vi "MH_RateDatAvg.vi"(0 "Rate Data":i32[][](array[numeric]), 1 "ClearRef":refnum<vi>, 3 "Avg ref":refnum<vi>, 5 "Count Rates":i32[](array[numeric]), 9 "RateAvg Data":i32[][](array[numeric]), 11 "error in (no error)":errorcluster caption="entrée d'erreur (pas d'erreur)", 12 "Avg Val":i32) -> (4 "Rate Data Out":i32[][](array[numeric]), 6 "Data":cluster{dbl, dbl, dbl, dbl}[](array[cluster]), 10 "RateAvg Data Out":i32[][](array[numeric]) format="%.2f", 13 "ValAvg":i32[](array[numeric]), 14 "Avg Val Out":i32, 15 "error out":errorcluster caption="sortie d'erreur")   [LabVIEW 2019]
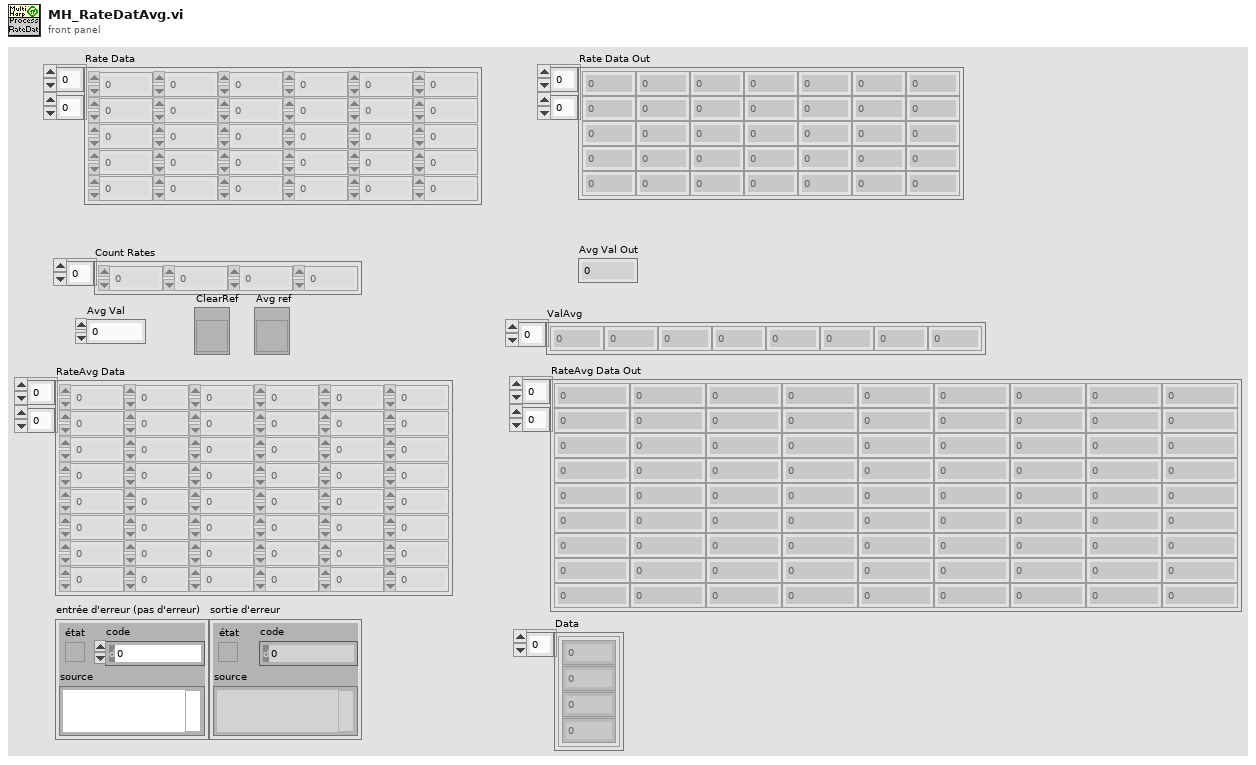
[diagram p1: front panel]
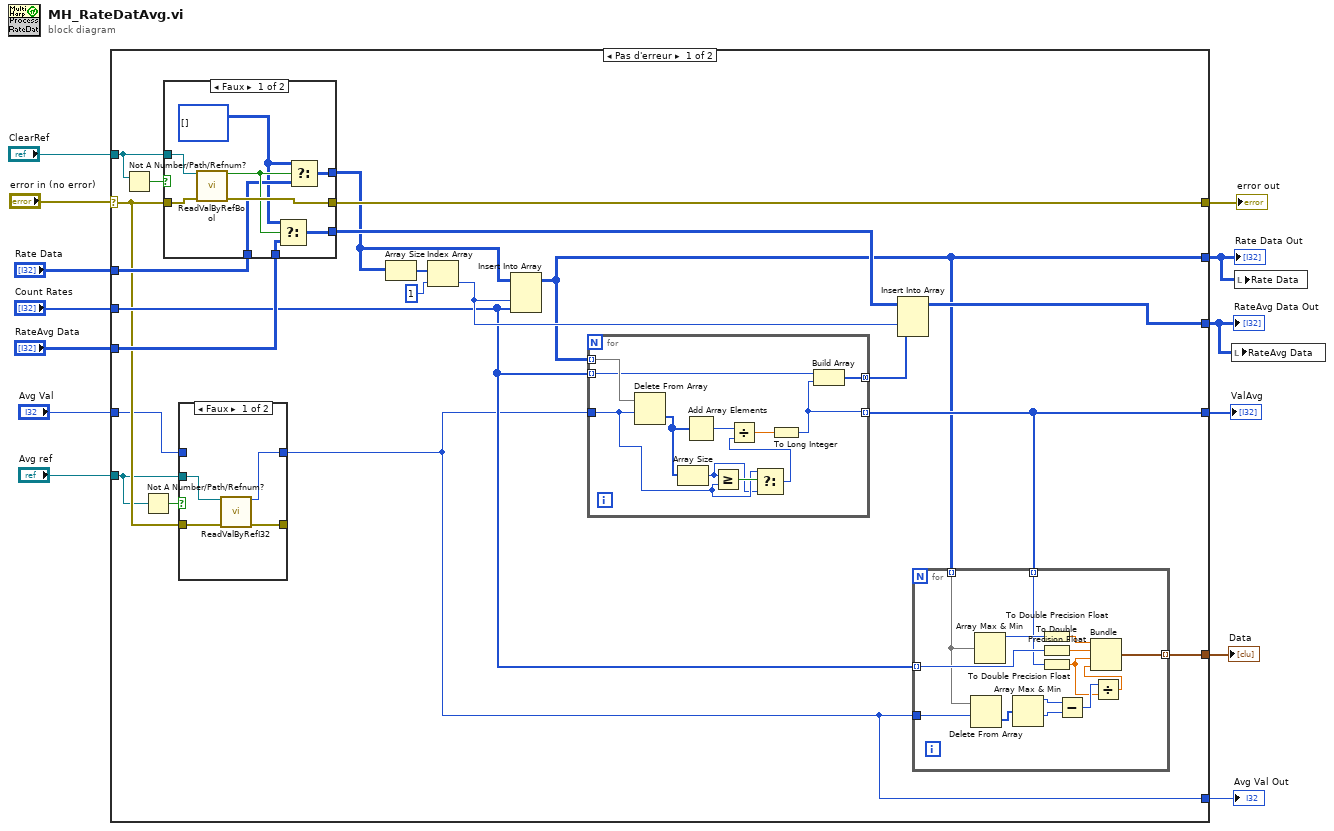
[diagram p0: block diagram]
diagram:
  n1 = case shown="Pas d'erreur" "error in (no error)" {
    selector: "error in (no error)" -> [w21 w80]
    tunnel: "Avg Val" -> [w18 _]
    tunnel: [w16 w79] -> w2
    tunnel: "Rate Data" -> [w26 w79]
    tunnel: "Count Rates" -> [w23 _]
    tunnel: "RateAvg Data" -> [w27 w78]
    tunnel: [w22 w78] -> w1
    tunnel: [w17 _] -> w9
    tunnel: [w30 w80] -> w7
    tunnel: "ClearRef" -> [w28 _]
    tunnel: "Avg ref" -> [w20 _]
    tunnel: [w15 _] -> w4
    tunnel: [w14 _] -> w3
    frame No Error {
      n2 = Not A Number/Path/Refnum?(number/path/refnum=w28) -> (NaN/Path/Refnum?=w29:bool)
      n3 = Not A Number/Path/Refnum?(number/path/refnum=w20) -> (NaN/Path/Refnum?=w19:bool)
      n4 = case shown="Faux" w29 {
        tunnel: w21 -> [w63 w66]
        tunnel: [w62 w66] -> w30
        tunnel: w28 -> [w61 _]
        tunnel: w27 -> [w58 w65]
        tunnel: w26 -> [w59 w64]
        tunnel: [w57 w65] -> w25
        tunnel: [w56 w64] -> w24
        frame False {
          w55 = i32[][] [] ("cas vrai")
          n5 = call <userlib>:"ReadValByRefBool.vi"("Control Ref"=w61, "error in"=w63) -> ("Valeur"=w60:bool, "error out"=w62:errorcluster)  [unwired: 12 in]
          n6 = Select(t=w55, s=w60, f=w58) -> (s? t:f=w57:i32[][])
          n7 = Select(t=w55, s=w60, f=w59) -> (s? t:f=w56:i32[][])
        }
        frame True {
        }
      }
      n8 = case shown="Faux" w19 {
        tunnel: w21 -> [w38 w40]
        tunnel: [w36 w40] -> _
        tunnel: w20 -> [w37 _]
        tunnel: w18 -> [_ w39]
        tunnel: [w35 w39] -> w14
        frame False {
          n9 = call <userlib>:"ReadValByRefI32.vi"("Control Ref"=w37, "error in"=w38) -> ("Valeur"=w35:i32, "error out"=w36:errorcluster)  [unwired: 12 in]
        }
        frame True {
        }
      }
      n10 = Array Size(array=w24) -> (size(s)=w34:i32[])
      n11 = Index Array(array=w34, index=1 ("indice")) -> (element=w32:i32)
      n12 = Insert Into Array(array=w24, index (col)=w32, new element=w23) -> (w16:i32[][])  [unwired: 1 in]
      n13 = for {
        tunnel: w16 -> [w77] mode=indexing
        tunnel: w14 -> [w70]
        tunnel: w23 -> [w74] mode=indexing
        tunnel: [w73] -> w31 mode=concatenating
        tunnel: [w67] -> w17 mode=indexing
        n14 = Delete From Array(array=w77, length=w70) -> (deleted portion=w72:i32[])  [unwired: 1 in, 1 out]
        n15 = Array Size(array=w72) -> (size(s)=w68:i32)
        n16 = Add Array Elements(numeric array=w72) -> (sum=w76:i32)
        n17 = Greater Or Equal?(x=w68, y=w70) -> (x >= y?=w71:bool)
        n18 = Select(t=w70, s=w71, f=w68) -> (s? t:f=w69:i32)
        n19 = Divide(x=w76, y=w69) -> (x/y=w75:dbl)
        n20 = To Long Integer(number=w75) -> (32bit integer=w67:i32)
        n21 = Build Array(w74, w67) -> (w73:i32[])
      }
      n22 = Insert Into Array(array=w25, index (col)=w32, new element=w31) -> (w22:i32[][])  [unwired: 1 in]
      n23 = for {
        tunnel: w16 -> [w49] mode=indexing
        tunnel: w23 -> [w51] mode=indexing
        tunnel: [w54] -> w15 mode=indexing
        tunnel: w14 -> [w48]
        tunnel: w17 -> [w41] mode=indexing
        n24 = Delete From Array(array=w49, length=w48) -> (deleted portion=w47:i32[])  [unwired: 1 in, 1 out]
        n25 = Array Max & Min(array=w49) -> (max value=w50:i32)  [unwired: 3 out]
        n26 = Array Max & Min(array=w47) -> (max value=w46:i32, min value=w45:i32)  [unwired: 2 out]
        n27 = To Double Precision Float(number=w50) -> (double precision float=w53:dbl)
        n28 = To Double Precision Float(number=w51) -> (double precision float=w52:dbl)
        n29 = To Double Precision Float(number=w41) -> (double precision float=w43:dbl)
        n30 = Subtract(x=w46, y=w45) -> (x-y=w44:i32)
        n31 = Divide(x=w44, y=w43) -> (x/y=w42:dbl)
        n32 = Bundle(w53, w52, w43, w42) -> (w54:cluster{dbl, dbl, dbl, dbl})  [unwired: 1 in]
      }
    }
    frame Error {
    }
  }
  "Rate Data Out" <- w2
  "RateAvg Data Out" <- w1
  "ValAvg" <- w9
  "error out" <- w7
  "Avg Val Out" <- w3
  "Data" <- w4
  n33 = local write "RateAvg Data"(w1) -> ()
  n34 = local write "Rate Data"(w2) -> ()
